vi "CAN Get Error Text.vi"(8 "error in (no error)":errorcluster caption="错误输入（无错误）", 9 "Buffer":string, 10 "Language":u16, 11 "Error":u32) -> (0 "error out":errorcluster caption="错误输出", 1 "Buffer out":string, 3 "function return":u32)   [LabVIEW 2017]
doc: "TPCANStatus __stdcall CAN_GetErrorText(\n TPCANStatus Error, \n WORD Language, \n LPSTR Buffer);"
uses:
  PCANBasic.dll
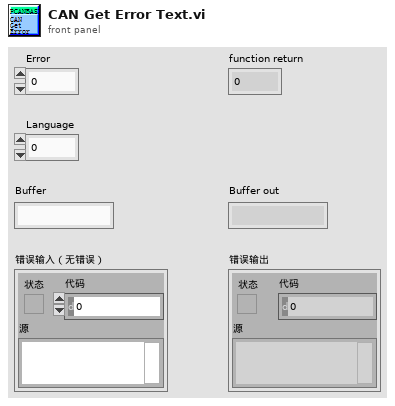
[diagram p1: front panel]
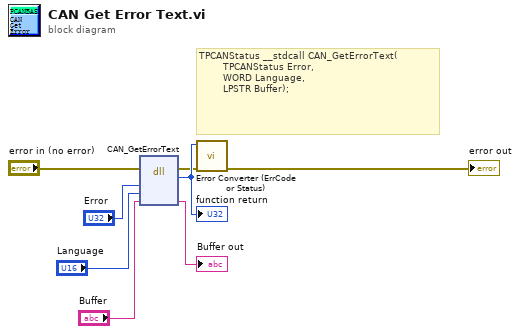
[diagram p0: block diagram]
diagram:
  # "TPCANStatus __stdcall CAN_GetErrorText(\n        TPCANStatus Error, \n        WORD Language, \n        LPSTR Buffer);"
  n1 = dll-call lib="PCANBasic.*" fn="CAN_GetErrorText"(error in="error in (no error)", "Error"="Error", "Language"="Language", "Buffer"="Buffer") -> (error out=w2:errorcluster, w8:u32, "Buffer"=→"Buffer out":string)  [unwired: 4 in, 1 out]
  "function return" <- w8
  n2 = call "Error Converter (ErrCode or Status).vi"("error in (no error)"=w2, "error code"=w8) -> ("error out"=→"error out":errorcluster)  [unwired: 9 in]
